vi "COMPARE CREDIT VS PRICE.vi"(7 "QUANTITY":i32, 8 "error in (no error)":errorcluster, 9 "PRICE":dbl, 10 "PRODUCT":string) -> (0 "error out":errorcluster)   [LabVIEW 2019, in "COINS.lvlib"]
doc: "HERE WE ARE GOING TO MAKE A COMPARISON OF OUR CREDIT AND THE PRICE OF THE PRODUCT SELECTED\n_____\nCreated using Delacor QMH Event Scripter 5.0.0.112."
uses:
  COINS.lvlib
  COMPARE CREDIT VS PRICE Argument--cluster.ctl
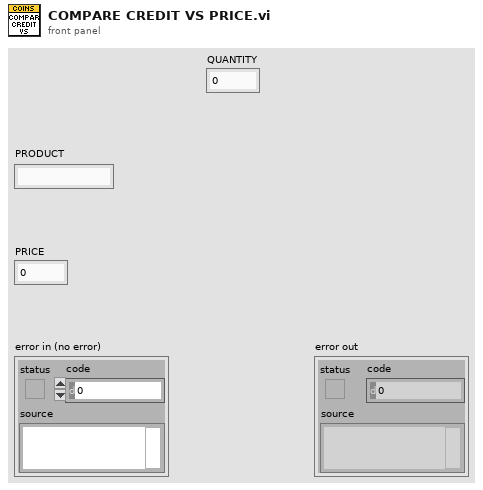
[diagram p1: front panel]
types:
  T1 = typedef "COINS.lvlib/COMPARE CREDIT VS PRICE Argument--cluster.ctl" = cluster{"PRODUCT":string, "PRICE":dbl, "QUANTITY":i32}
  T2 = typedef "COINS.lvlib/Request Events--cluster.ctl" = cluster{"Stop Module":refnum<user-event>, "Show Panel":refnum<user-event>, "Hide Panel":refnum<user-event>, "Get Module Execution Status":refnum<user-event>, "Show Diagram":refnum<user-event>, "SET COINS":refnum<user-event>, "UPDATE COIN":refnum<user-event>, "UPDATE CREDIT":refnum<user-event>, "COMPARE CREDIT VS PRICE":refnum<user-event>}
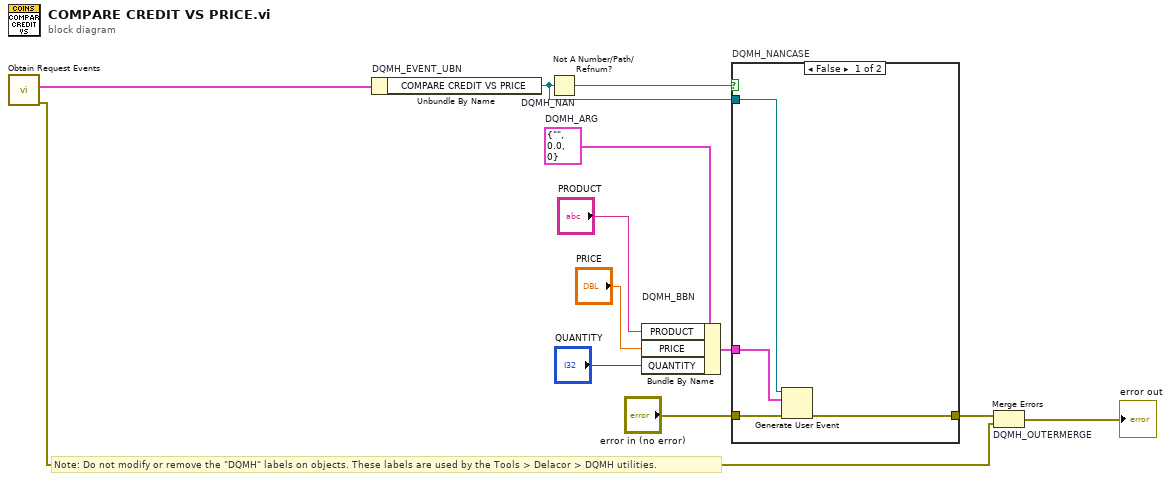
[diagram p0: block diagram]
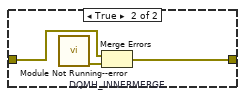
[diagram p2: hidden frame]
diagram:
  w6 = T1 {"PRODUCT"="", "PRICE"=0.0, "QUANTITY"=0}  # DQMH_ARG
  # "Note: Do not modify or remove the \"DQMH\" labels on objects. These labels are used by the Tools > Delacor > DQMH utilities."
  n1 = call "Obtain Request Events.vi"() -> ("error out"=w2:errorcluster, "COINS Request Events"=w1:T2)  [unwired: 10 in]
  n2 = Unbundle By Name "DQMH_EVENT_UBN"(w1) -> ("COMPARE CREDIT VS PRICE"=w8:refnum<user-event>)
  n3 = Not A Number/Path/Refnum? "DQMH_NAN"(number/path/refnum=w8) -> (NaN/Path/Refnum?=w9:bool)
  n4 = Bundle By Name "DQMH_BBN"(cluster=w6, "PRODUCT"="PRODUCT", "PRICE"="PRICE", "QUANTITY"="QUANTITY") -> (w10:T1)
  n5 = case "DQMH_NANCASE" shown="False" w9 {
    tunnel: "error in (no error)" -> [w16 w19]
    tunnel: [w15 w18] -> w7
    tunnel: w8 -> [w14 _]
    tunnel: w10 -> [w13 _]
    frame False {
      n6 = Generate User Event(user event=w14, event data cluster=w13, error in=w16) -> (error out=w15:errorcluster)  [unwired: 1 in, 1 out]
    }
    frame True {
      n7 = call "Module Not Running--error.vi"() -> ("error out"=w17:errorcluster)  [unwired: 11 in]
      n8 = Merge Errors "DQMH_INNERMERGE"(w19, w17) -> (w18:errorcluster)
    }
  }
  n9 = Merge Errors "DQMH_OUTERMERGE"(w7, w2) -> (→"error out":errorcluster)
